vi "Example Main.vi"() -> ()   [LabVIEW 2014]
uses:
  DataGridView/DataGridView.lvclass
  GridColumn/GridColumn.lvclass
  System.Windows.Forms
panel:
  in  "DataGridView":refnum<k24>(container)
  out "code":i32
  out "status":bool
  out "Error Source":string
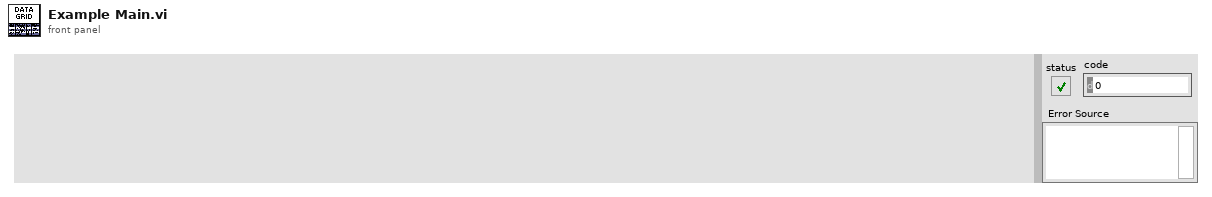
[diagram p1: front panel]
types:
  T1 = cluster{"Name":string, "Link":string, "Created By":string, "Action":string, "Type":enum16{"ONE", "TWO", "THREE"}, "Comments":string, "Active":bool, "Image":string}[]
  T2 = cluster{"name":string, "datatype":enum16{"string", "image", "link", "check", "combo", "button"}, "Params":string, "AutoSizeMode":i32, "FillWeight":sgl, "AutoSizeMode 2":i32}[]
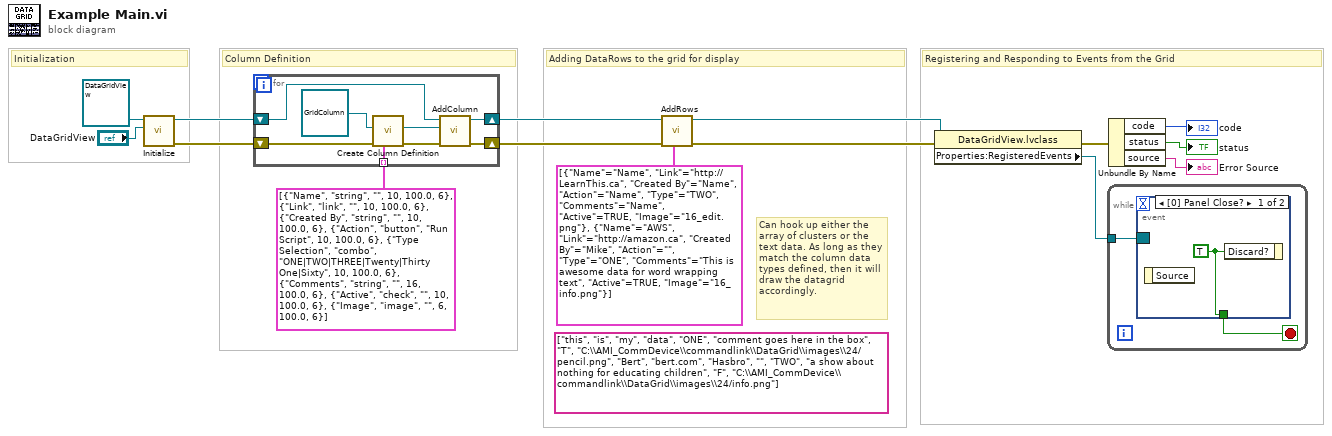
[diagram p0: block diagram]
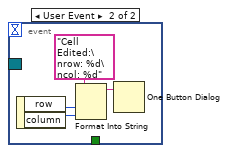
[diagram p2: hidden frame]
diagram:
  (unwired) string[][] [["this", "is", "my", "data", "ONE", "comment goes here in the box", "T", "C:\\AMI_CommDevice\\commandlink\\DataGrid\\images\\24/pencil.png"], ["Bert", "bert.com", "Hasbro", "", "TWO", "a show about nothing for educating children", "F", "C:\\AMI_CommDevice\\commandlink\\DataGrid\\images\\24/info.png"]]
  # "Registering and Responding to Events from the Grid"
  # "Adding DataRows to the grid for display"
  # "Column Definition"
  # "Initialization"
  # "Can hook up either the array of clusters or the text data. As long as they match the column data types defined, then it will draw the datagrid accordingly."
  n1 = call "Initialize.vi"("DataGridView"="DataGridView", "DataGrid in"=refnum<class "DataGridView.lvclass"> refnum ("DataGrid.lvclass")) -> ("error out"=w13:errorcluster, "DataGrid out"=w14:refnum<class "DataGridView.lvclass">)  [unwired: 8 in]
  n2 = for {
    shift-right: [w22] -> w11
    shift-left: w14 -> [w23]
    shift-right: [w19] -> w12
    shift-left: w13 -> [w20]
    tunnel: T2 [{"name"="Name", "datatype"=enum."string", "Params"="", "AutoSizeMode"=10, "FillWeight"=100.0, "AutoSizeMode 2"=6}, {"name"="Link", "datatype"=enum."link", "Params"="", "AutoSizeMode"=10, "FillWeight"=100.0, "AutoSizeMode 2"=6}, {"name"="Created By", "datatype"=enum."string", "Params"="", "AutoSizeMode"=10, "FillWeight"=100.0, "AutoSizeMode 2"=6}, {"name"="Action", "datatype"=enum."button", "Params"="Run Script", "AutoSizeMode"=10, "FillWeight"=100.0, "AutoSizeMode 2"=6}, {"name"="Type Selection", "datatype"=enum."combo", "Params"="ONE|TWO|THREE|Twenty|Thirty One|Sixty", "AutoSizeMode"=10, "FillWeight"=100.0, "AutoSizeMode 2"=6}, {"name"="Comments", "datatype"=enum."string", "Params"="", "AutoSizeMode"=16, "FillWeight"=100.0, "AutoSizeMode 2"=6}, {"name"="Active", "datatype"=enum."check", "Params"="", "AutoSizeMode"=10, "FillWeight"=100.0, "AutoSizeMode 2"=6}, {"name"="Image", "datatype"=enum."image", "Params"="", "AutoSizeMode"=6, "FillWeight"=100.0, "AutoSizeMode 2"=6}] -> [w16] mode=indexing
    n3 = call "Create Column Definition.vi"("Column Definition"=w16, "error in (no error)"=w20, "GridColumn in"=refnum<class "GridColumn.lvclass"> refnum ("GridColumn.lvclass")) -> ("error out"=w21:errorcluster, "GridColumn out"=w18:refnum<class "GridColumn.lvclass">)  [unwired: 7 in]
    n4 = call "AddColumn.vi"("error in (no error)"=w21, "GridColumn.lvclass"=w18, "DataGrid in"=w23) -> ("error out"=w19:errorcluster, "DataGrid out"=w22:refnum<class "DataGridView.lvclass">)  [unwired: 7 in]
  }
  n5 = call "AddRows.vi"("GridData"=T1 [{"Name"="Name", "Link"="http://LearnThis.ca", "Created By"="Name", "Action"="Name", "Type"=enum."TWO", "Comments"="Name", "Active"=TRUE, "Image"="16_edit.png"}, {"Name"="AWS", "Link"="http://amazon.ca", "Created By"="Mike", "Action"="", "Type"=enum."ONE", "Comments"="This is awesome data for word wrapping text", "Active"=TRUE, "Image"="16_info.png"}], "error in (no error)"=w12, "DataGridView in"=w11) -> ("error out"=w3:errorcluster, "DataGridView out"=w4:refnum<class "DataGridView.lvclass">)  [unwired: 7 in]
  n6 = property class="DataGridView.lvclass"(reference=w4, error in=w3) -> (error out=w2:errorcluster, "Properties:RegisteredEvents"=w1:refnum<event-registration>)  [unwired: 1 out]
  n7 = while {
    tunnel: w1 -> [w25]
    stop <- w24 stop-if-true
    n8 = event shown="[0] Panel Close?" {
      selector: w25 -> [_ _]
      dyn-events: _ -> [_ _]
      timeout: _ -> [_ _]
      tunnel: [w26 _] -> w24
      event Panel Close? {
        w26 = TRUE ("Discard?")
        n9 = event-data() -> ()  [unwired: 1 in, 1 out]
        n10 = event-data("Discard?"=w26) -> ()  [unwired: 1 in, 1 out]
      }
      event User Event {
        n11 = event-data() -> ("row"=w27:i32, "column"=w28:i32)  [unwired: 1 in]
        n12 = Format Into String(format string="Cell Edited:\nrow: %d\ncol: %d" ("message"), w27, w28) -> (resulting string=w30:string)  [unwired: 2 in, 1 out]
        n13 = One Button Dialog(message=w30) -> ()  [unwired: 1 in, 1 out]
      }
    }
  }
  n14 = Unbundle By Name(w2) -> ("code"=→"code":i32, "status"=→"status":bool, "source"=→"Error Source":string)
